vi "Save and Load VI State.vi"() -> ()   [LabVIEW 2015]
doc: "Example VI that demonstrates VI state saving and loading."
uses:
  PL Utility.lvlib
panel:
  in  "load":bool
  in  "save":bool
  out "indicator":dbl
  in  "control":dbl
  in  "stop":bool
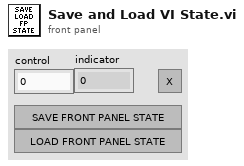
[diagram p1: front panel]
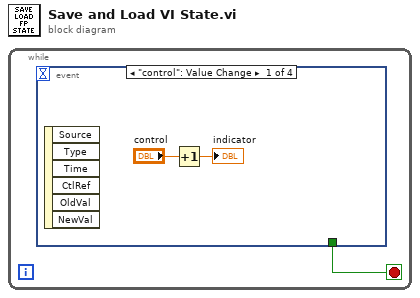
[diagram p0: block diagram]
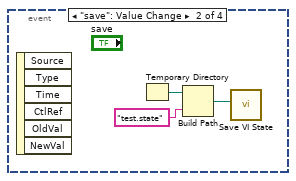
[diagram p2: hidden frame]
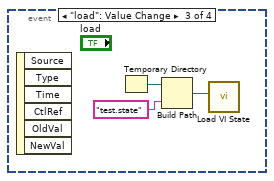
[diagram p3: hidden frame]
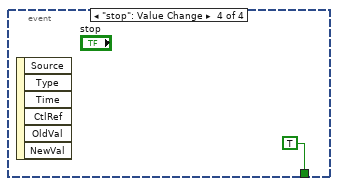
[diagram p4: hidden frame]
diagram:
  n1 = while {
    stop <- w1 stop-if-true
    n2 = event shown="[0] \"control\": Value Change" {
      selector: _ -> [_ _ _ _]
      dyn-events: _ -> [_ _ _ _]
      timeout: _ -> [_ _ _ _]
      tunnel: [_ _ _ TRUE] -> w1
      event "control": Value Change {
        n3 = event-data() -> ()  [unwired: 1 in, 6 out]
        n4 = Increment(x="control") -> (x+1=→"indicator":dbl)
      }
      event "save": Value Change {
        n5 = event-data() -> ()  [unwired: 1 in, 6 out]
        n6 = Temporary Directory() -> (w5:path)
        n7 = Build Path(base path=w5, name or relative path="test.state") -> (appended path=w4:path)
        n8 = call "Save VI State.vi"("state file path (<application path>\\<vi name>.state)"=w4) -> ()  [unwired: 10 in, 1 out]
      }
      event "load": Value Change {
        n9 = event-data() -> ()  [unwired: 1 in, 6 out]
        n10 = Temporary Directory() -> (w8:path)
        n11 = Build Path(base path=w8, name or relative path="test.state") -> (appended path=w7:path)
        n12 = call "Load VI State.vi"("state file path (<application path>\\<vi name>.state)"=w7) -> ()  [unwired: 10 in, 1 out]
      }
      event "stop": Value Change {
        n13 = event-data() -> ()  [unwired: 1 in, 6 out]
      }
    }
  }
